vi "Square waveform.vi"() -> ()   [LabVIEW 2020]
uses:
  <vilib>/DAQmx/write.llb/DAQmx Write (Analog Wfm 1Chan NSamp).vi
  <vilib>/DAQmx/create/channels.llb/DAQmx Create Channel (AO-Voltage-Basic).vi
  <vilib>/DAQmx/configure/timing.llb/DAQmx Timing (Sample Clock).vi
  <vilib>/DAQmx/miscellaneous.llb/DAQmx Fill In Error Info.vi
  <vilib>/measure/NI_MABase.lvlib
panel:
  out "number of samples written per channel":u32
  in  "stop":bool
  in  "offset":dbl format="%.2p"
  out "Waveform Graph":waveform(dbl)(graph)
  in  "phase":dbl format="%.2p"
  in  "amplitude":dbl=1.0 format="%.2p"
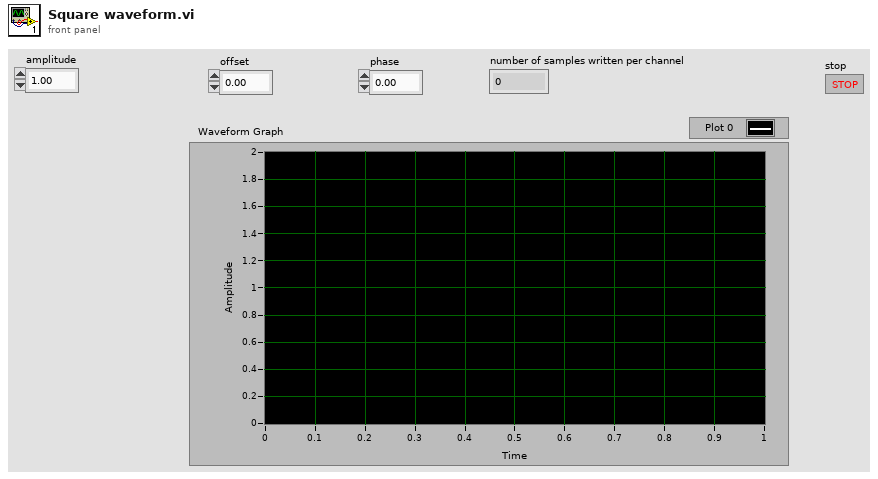
[diagram p1: front panel]
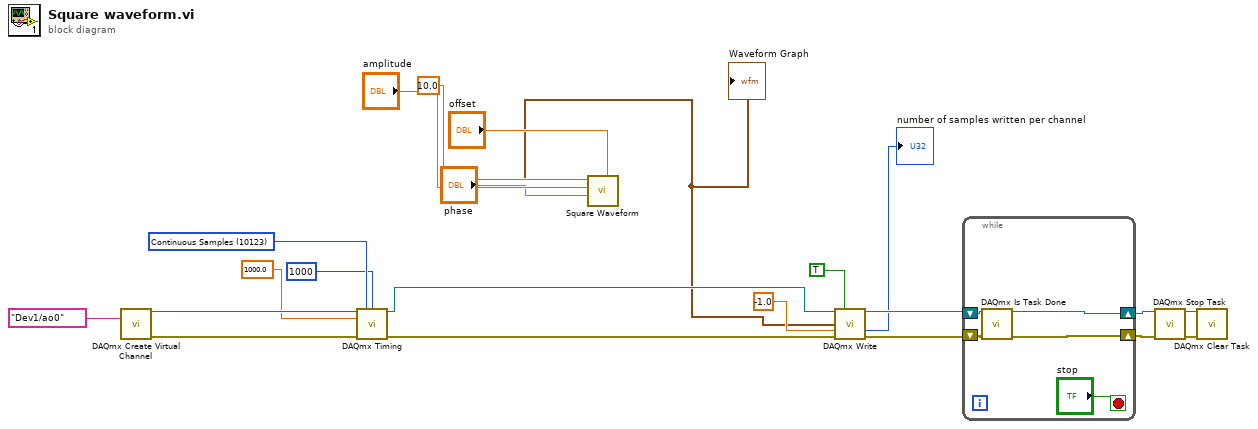
[diagram p0: block diagram]
diagram:
  w15 = 10123 items=["Finite Samples"=10178, "Continuous Samples"=10123, "Hardware Timed Single Point"=12522] ("sample mode")
  n1 = call-poly <vilib>:"DAQmx Create Virtual Channel.vi"("physical channels"=tag "Dev1/ao0") -> ("task out"=w17:refnum<k21>, "error out"=w16:errorcluster)  [unwired: 13 in]
  n2 = call-poly <vilib>:"DAQmx Timing.vi"("task/channels in"=w17, "sample mode"=w15, "samples per channel"=1000, "rate"=1000.0, "error in"=w16) -> ("task out"=w9:refnum<k21>, "error out"=w8:errorcluster)  [unwired: 9 in]
  n3 = call <vilib>:"Square Waveform.vi"("offset"="offset", "phase"="phase", "amplitude"="amplitude", "frequency"=10.0) -> ("signal out"=w1:waveform(dbl))  [unwired: 6 in, 1 out]
  "Waveform Graph" <- w1
  n4 = call-poly <vilib>:"DAQmx Write.vi"("task/channels in"=w9, "auto start"=TRUE, "data"=w1, "timeout"=-1.0, "error in"=w8) -> ("task out"=w12:refnum<k21>, "number of samples written per channel"=→"number of samples written per channel":u32, "error out"=w13:errorcluster)  [unwired: 8 in]
  n5 = while {
    shift-right: [w24] -> w4
    shift-left: w12 -> [w27]
    shift-right: [w25] -> w5
    shift-left: w13 -> [w26]
    stop <- "stop" stop-if-true
    n6 = call <vilib>:"DAQmx Is Task Done.vi"("task/channels in"=w27, "error in"=w26) -> ("task out"=w24:refnum<k21>, "error out"=w25:errorcluster)  [unwired: 11 in, 1 out]
  }
  n7 = call <vilib>:"DAQmx Stop Task.vi"("task/channels in"=w4, "error in"=w5) -> ("task out"=w19:refnum<k21>, "error out"=w20:errorcluster)  [unwired: 12 in]
  n8 = call <vilib>:"DAQmx Clear Task.vi"("task in"=w19, "error in"=w20) -> ()  [unwired: 13 in, 1 out]
